vi "DAQ-Enumerate COM Ports.vi"() -> (8 "COM ports":string[](array[string]))   [LabVIEW 2020]
uses:
  <vilib>/Instr/_visa.llb/VISA Find Search Mode.ctl
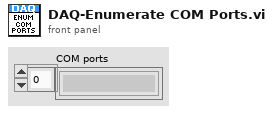
[diagram p1: front panel]
types:
  T1 = typedef "VISA Find Search Mode.ctl" = u32
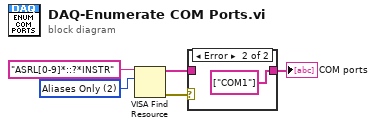
[diagram p0: block diagram]
diagram:
  w2 = T1 2 items=["Canonical Names Only"=0, "Aliases Only"=2, "Include Matching Aliases"=3, "Include All Aliases"=4] ("Search Mode")
  n1 = VISA Find Resource(10:w2, 11:"ASRL[0-9]*::?*INSTR" ("expression (\"?*\")")) -> (0:w5:errorcluster, 3:w4:string[])  [unwired: 1 in, 1 out]
  n2 = case shown="Error" w5 {
    tunnel: w4 -> [w6 _]
    tunnel: [w6 string[] ["COM1"] ("find list")] -> w1
    frame No Error {
    }
    frame Error {
    }
  }
  "COM ports" <- w1
